vi "Update UI per Reference.vi"(8 "error in (no error)":errorcluster, 11 "Analyze Results Fluence and Energy in":refnum<class "Analyze Results Fluence and Energy.lvclass">) -> (0 "error out":errorcluster, 3 "Analyze Results Fluence and Energy out":refnum<class "Analyze Results Fluence and Energy.lvclass">)   [LabVIEW 2014, in "Analyze Results Fluence and Energy.lvclass"]
uses:
  Analyze Results Fluence and Energy.lvclass
  Analyze Results Fluence and Energy.lvclass/Analyze Results Fluence and Energy.ctl
  JETI200 Overview and ShotID/HIJ Vision/Analyze/Results and Overlays/Results Base/Analyze Results Base.lvclass
  JETI200 Overview and ShotID/HIJ Vision/Analyze/Results and Overlays/Results Energy/Analyze Results Energy.lvclass
  JETI200 Overview and ShotID/HIJ Vision/Analyze/Results and Overlays/Results Fluence/Analyze Results Fluence.lvclass
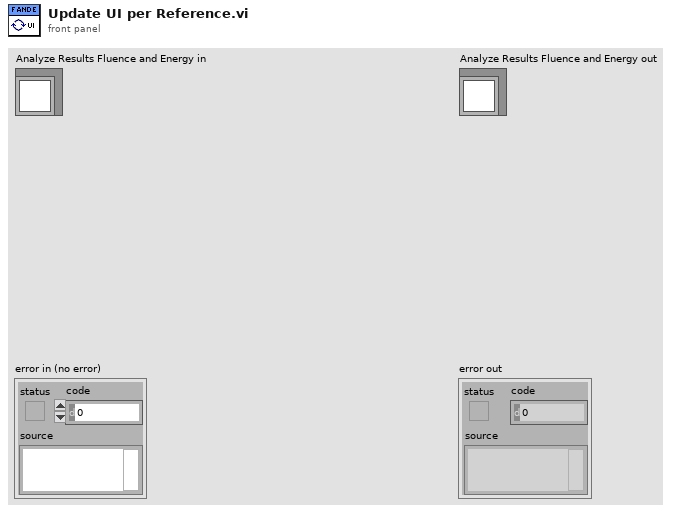
[diagram p1: front panel]
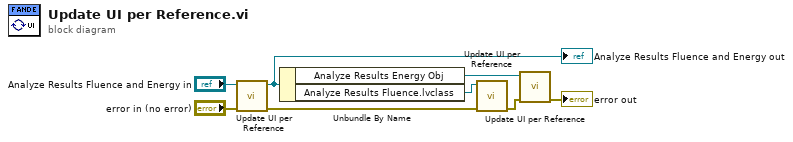
[diagram p0: block diagram]
diagram:
  n1 = call-parent "Update UI per Reference.vi"("error in (no error)"="error in (no error)", "Analyze Results Base in"="Analyze Results Fluence and Energy in") -> ("error out"=w2:errorcluster, "Analyze Results Base out"=w6:refnum<class "Analyze Results Fluence and Energy.lvclass">)  [unwired: 8 in]
  "Analyze Results Fluence and Energy out" <- w6
  n2 = Unbundle By Name(w6) -> ("Analyze Results Energy Obj"=w5:refnum<class "Analyze Results Energy.lvclass">, "Analyze Results Fluence.lvclass"=w4:refnum<class "Analyze Results Fluence.lvclass">)
  n3 = call-dynamic "Update UI per Reference.vi"("error in (no error)"=w2, "Analyze Results Fluence in"=w4) -> ("error out"=w3:errorcluster)  [unwired: 8 in, 1 out]
  n4 = call-dynamic "Update UI per Reference.vi"("error in (no error)"=w3, "Analyze Results Energy in"=w5) -> ("error out"=→"error out":errorcluster)  [unwired: 8 in, 1 out]
